vi "WLAN - TV - RW - ReadTestVectorFile(Tx) dll.vi"(0 "file path (dialog if empty)":path, 5 "TestItem_Index":i32) -> (4 "TV's":T1[](array[typedef]) {"Tx_Chan" format="%.0x"; "Standard" items=["80211A/G/J/P OFDM", "80211B/G DSSS", "80211G DSSSOFDM", "80211N MIMOOFDM", "80211AC MIMOOFDM"]; "OFDM Data Rate (Mbps)" items=["6", "9", "12", "18", "24", "36", "48", "54"]; "80211n PLCP Frame Format" items=["Mixed Format", "Greenfield Format"]; "FEC Coding Type" items=["BCC", "LDPC"]; "DSSS Data Rate (Mbps)" items=["1", "2", "5.5 CCK", "5.5 PBCC", "11 CCK", "11 PBCC", "22", "33"]}, 6 "Tv First Element":T1 {"Tx_Chan" format="%.0x"; "Standard" items=["80211A/G/J/P OFDM", "80211B/G DSSS", "80211G DSSSOFDM", "80211N MIMOOFDM", "80211AC MIMOOFDM"]; "OFDM Data Rate (Mbps)" items=["6", "9", "12", "18", "24", "36", "48", "54"]; "80211n PLCP Frame Format" items=["Mixed Format", "Greenfield Format"]; "FEC Coding Type" items=["BCC", "LDPC"]; "DSSS Data Rate (Mbps)" items=["1", "2", "5.5 CCK", "5.5 PBCC", "11 CCK", "11 PBCC", "22", "33"]}, 8 "Current TV Element":T1 {"Tx_Chan" format="%.0x"; "Standard" items=["80211A/G/J/P OFDM", "80211B/G DSSS", "80211G DSSSOFDM", "80211N MIMOOFDM", "80211AC MIMOOFDM"]; "OFDM Data Rate (Mbps)" items=["6", "9", "12", "18", "24", "36", "48", "54"]; "80211n PLCP Frame Format" items=["Mixed Format", "Greenfield Format"]; "FEC Coding Type" items=["BCC", "LDPC"]; "DSSS Data Rate (Mbps)" items=["1", "2", "5.5 CCK", "5.5 PBCC", "11 CCK", "11 PBCC", "22", "33"]})   [LabVIEW 2011]
uses:
  Includes/WLAN - TV - RW - INC - TV_DataType_Cluster.ctl
  Includes/WLAN - TV - RW - INC - TV_Parameters.ctl
  <vilib>/Utility/file.llb/Read From Spreadsheet File (string).vi
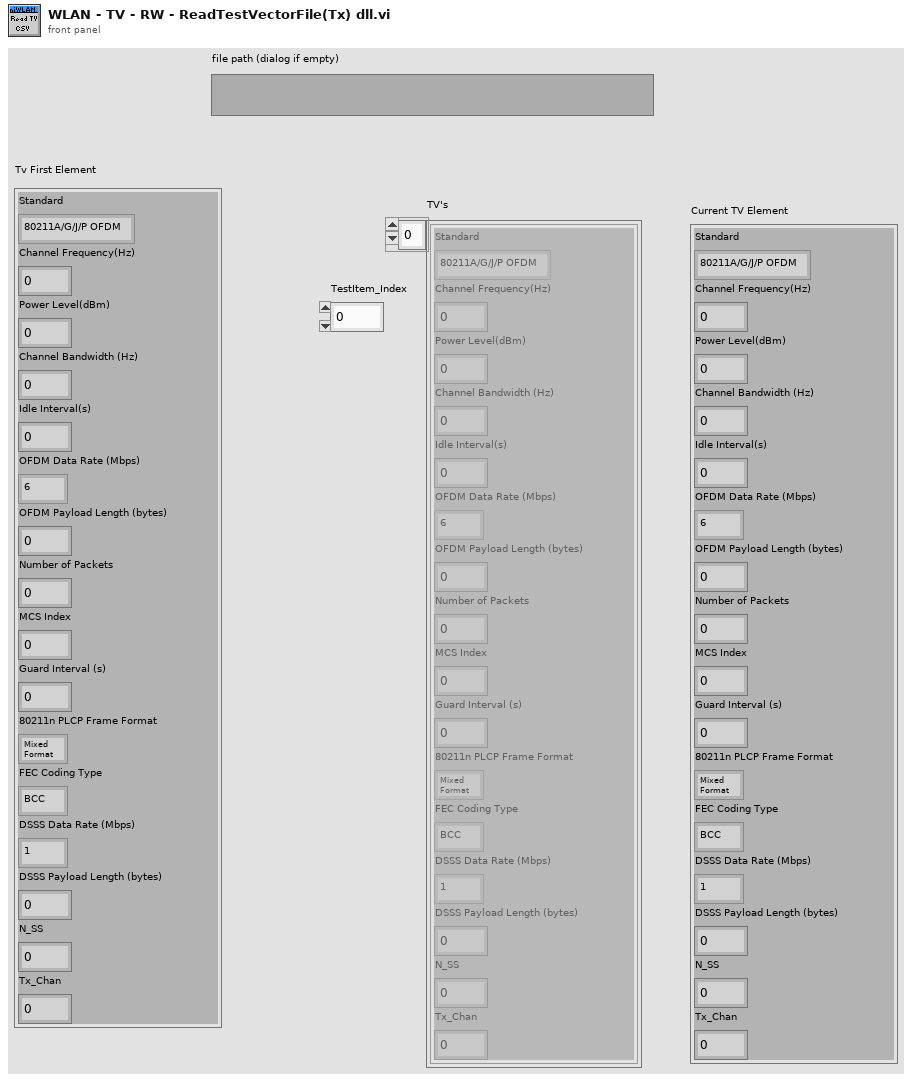
[diagram p1: front panel]
types:
  T1 = typedef "WLAN - TV - RW - INC - TV_DataType_Cluster.ctl" = cluster{"Standard":i32, "Channel Frequency(Hz)":dbl, "Power Level(dBm)":dbl, "Channel Bandwidth (Hz)":dbl, "Idle Interval(s)":dbl, "OFDM Data Rate (Mbps)":i32, "OFDM Payload Length (bytes)":i32, "Number of Packets":i32, "MCS Index":i32, "Guard Interval (s)":dbl, "80211n PLCP Frame Format":i32, "FEC Coding Type":i32, "DSSS Data Rate (Mbps)":i32, "DSSS Payload Length (bytes)":i32, "N_SS":i32, "Tx_Chan":u32}
  T2 = typedef "WLAN - TV - RW - INC - TV_Parameters.ctl" = cluster{"Standard ":string, "Channel Frequency(Hz)":string, "Power Level(dBm)":string, "Channel Bandwidth (Hz)":string, "Idle Interval (s)":string, "OFDM Data Rate (Mbps)":string, "OFDM Payload Length (bytes)":string, "MCS Index":string, "Guard Interval (s)":string, "80211n PLCP Frame Format":string, "FEC Coding Type":string, "DSSS Data Rate (Mbps)":string, "DSSS Payload Length (bytes)":string, "#Packets":string, "N_SS":string, "Tx_Chan":string}
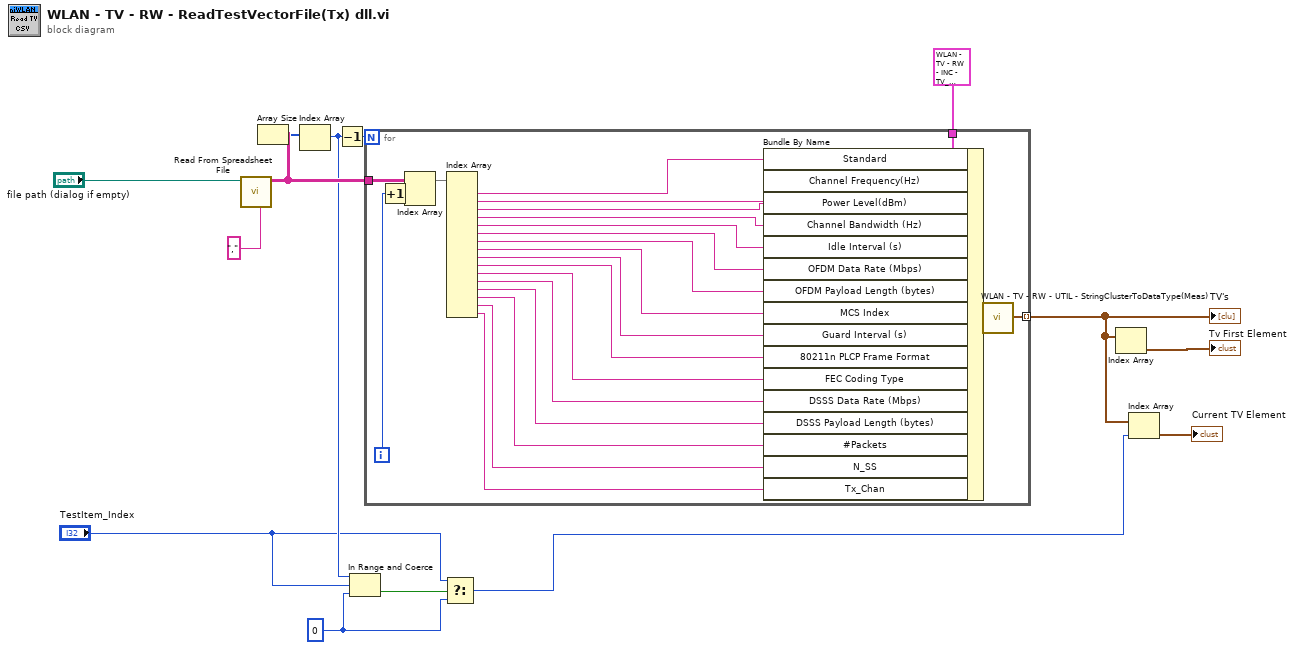
[diagram p0: block diagram]
diagram:
  w3 = 0 ("lower limit")
  n1 = call-poly <vilib>:"Read From Spreadsheet File.vi"("delimiter (\\t)"="," ("delimiter (\\t)"), "file path (dialog if empty)"="file path (dialog if empty)") -> ("all rows"=w10:string[][])  [unwired: 5 in, 4 out]
  n2 = Array Size(array=w10) -> (size(s)=w6:i32[])
  n3 = Index Array(array=w6) -> (element=w5:i32)  [unwired: 1 in]
  n4 = Decrement(x=w5) -> (x-1=w11:i32)
  n5 = In Range and Coerce(upper limit=w5, x="TestItem_Index", lower limit=w3) -> (In Range?=w4:bool)  [unwired: 1 out]
  n6 = for {
    N: w11 -> [_]
    tunnel: T2 {"Standard "="", "Channel Frequency(Hz)"="", "Power Level(dBm)"="", "Channel Bandwidth (Hz)"="", "Idle Interval (s)"="", "OFDM Data Rate (Mbps)"="", "OFDM Payload Length (bytes)"="", "MCS Index"="", "Guard Interval (s)"="", "80211n PLCP Frame Format"="", "FEC Coding Type"="", "DSSS Data Rate (Mbps)"="", "DSSS Payload Length (bytes)"="", "#Packets"="", "N_SS"="", "Tx_Chan"=""} ("TV Paramaters") -> [w37]
    tunnel: [w21] -> w8 mode=indexing
    tunnel: w10 -> [w20]
    i -> [w18]
    n7 = Increment(x=w18) -> (x+1=w17:i32)
    n8 = Index Array(array=w20, index (row)=w17) -> (element=w19:string[])  [unwired: 1 in]
    n9 = Index Array(array=w19) -> (element #1=w36:string, element #2=w35:string, element #3=w34:string, element #4=w33:string, element #5=w32:string, element #6=w31:string, element #7=w30:string, element #8=w29:string, element #9=w28:string, element #10=w27:string, element #11=w26:string, element #12=w25:string, element #13=w24:string, element #14=w23:string, element #15=w16:string, element #16=w15:string)  [unwired: 16 in]
    n10 = Bundle By Name(cluster=w37, "Standard"=w36, "Channel Frequency(Hz)"=w35, "Power Level(dBm)"=w34, "Channel Bandwidth (Hz)"=w33, "Idle Interval (s)"=w32, "OFDM Data Rate (Mbps)"=w31, "OFDM Payload Length (bytes)"=w30, "MCS Index"=w29, "Guard Interval (s)"=w28, "80211n PLCP Frame Format"=w27, "FEC Coding Type"=w26, "DSSS Data Rate (Mbps)"=w25, "DSSS Payload Length (bytes)"=w24, "#Packets"=w23, "N_SS"=w16, "Tx_Chan"=w15) -> (w22:T2)
    n11 = call "WLAN - TV - RW - UTIL - StringClusterToDataType(Meas).vi"("TV Paramaters(String)"=w22) -> ("TV Parameters(DataType)"=w21:T1)  [unwired: 14 in]
  }
  "TV's" <- w8
  n12 = Select(t="TestItem_Index", s=w4, f=w3) -> (s? t:f=w1:i32)
  n13 = Index Array(array=w8) -> (element=→"Tv First Element":T1)  [unwired: 1 in]
  n14 = Index Array(array=w8, index=w1) -> (element=→"Current TV Element":T1)
